vi "Set Cluster Values from ClusterRef.vi"(8 "error in":errorcluster, 10 "Target Cluster Ref":refnum<vi>, 11 "Source Cluster Ref":refnum<vi>) -> (0 "error out":errorcluster)   [LabVIEW 2023]
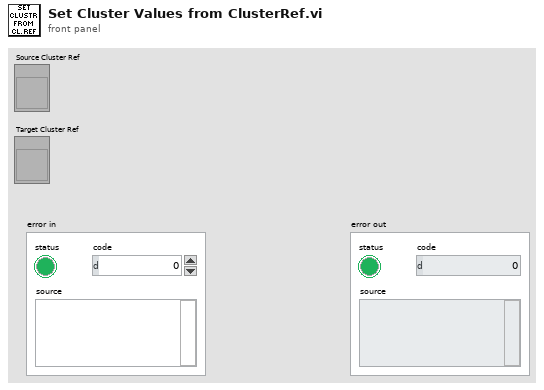
[diagram p1: front panel]
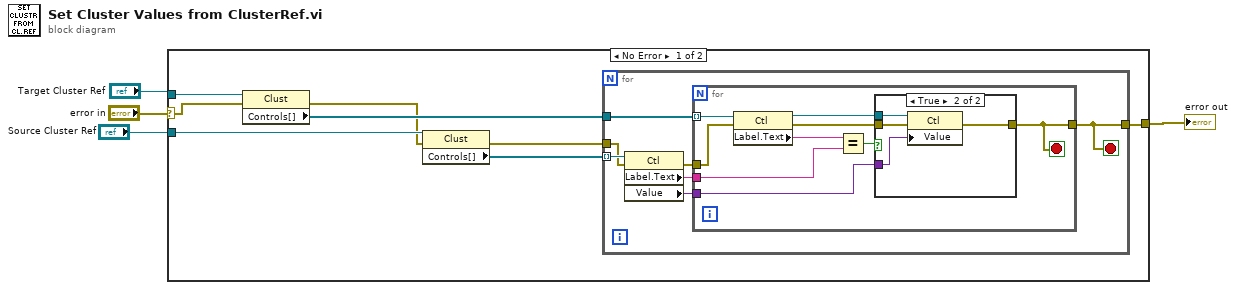
[diagram p0: block diagram]
diagram:
  n1 = case shown="No Error" "error in" {
    selector: "error in" -> [w6 w34]
    tunnel: "Source Cluster Ref" -> [w7 _]
    tunnel: [w8 w34] -> w3
    tunnel: "Target Cluster Ref" -> [w10 _]
    frame No Error {
      n2 = property class="Clust"(reference=w10, error in=w6) -> (error out=w5:errorcluster, "Controls[]"=w9:refnum<vi>[])  [unwired: 1 out]
      n3 = property class="Clust"(reference=w7, error in=w5) -> (error out=w11:errorcluster, "Controls[]"=w12:refnum<vi>[])  [unwired: 1 out]
      n4 = for {
        tunnel: w12 -> [w19] mode=indexing
        tunnel: w11 -> [w16]
        tunnel: w9 -> [w18]
        tunnel: [w13] -> w8
        stop <- w13 stop-if-true
        n5 = property class="Ctl"(reference=w19, error in=w16) -> (error out=w15:errorcluster, "Label.Text"=w17:string, "Value"=w14:variant)  [unwired: 1 out]
        n6 = for {
          tunnel: w18 -> [w28] mode=indexing
          tunnel: w17 -> [w26]
          tunnel: w15 -> [w25]
          tunnel: w14 -> [w22]
          tunnel: [w20] -> w13
          stop <- w20 stop-if-true
          n7 = property class="Ctl"(reference=w28, error in=w25) -> (reference out=w23:refnum<vi>, error out=w21:errorcluster, "Label.Text"=w27:string)
          n8 = Equal?(x=w27, y=w26) -> (x = y?=w24:bool)
          n9 = case shown="True" w24 {
            tunnel: w23 -> [_ w33]
            tunnel: w22 -> [_ w32]
            tunnel: w21 -> [w29 w31]
            tunnel: [w29 w30] -> w20
            frame False {
            }
            frame True {
              n10 = property class="Ctl"(reference=w33, error in=w31, "Value"=w32) -> (error out=w30:errorcluster)  [unwired: 1 out]
            }
          }
        }
      }
    }
    frame Error {
    }
  }
  "error out" <- w3
